vi "formatEvtDetails.vi"(8 "error in (no error)":errorcluster, 9 "evtName":string="move", 10 "evtDetailsString":string, 11 "TcpServer.lvclass":refnum<class "TcpServer.lvclass">) -> (0 "error out":errorcluster, 2 "jsonString":string, 3 "TcpServer.lvclass":refnum<class "TcpServer.lvclass">)   [LabVIEW 2018, in "TcpServer.lvclass"]
doc: "Prepare the Event with JSON format."
uses:
  TcpServer.lvclass
  <vilib>/Utility/error.llb/Error Cluster From Error Code.vi
  <vilib>/ErrorRing/Error Ring.xnode
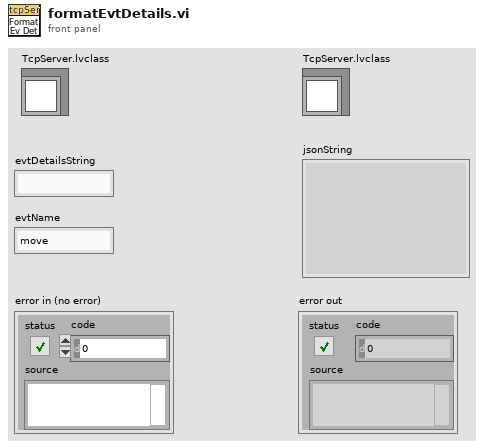
[diagram p1: front panel]
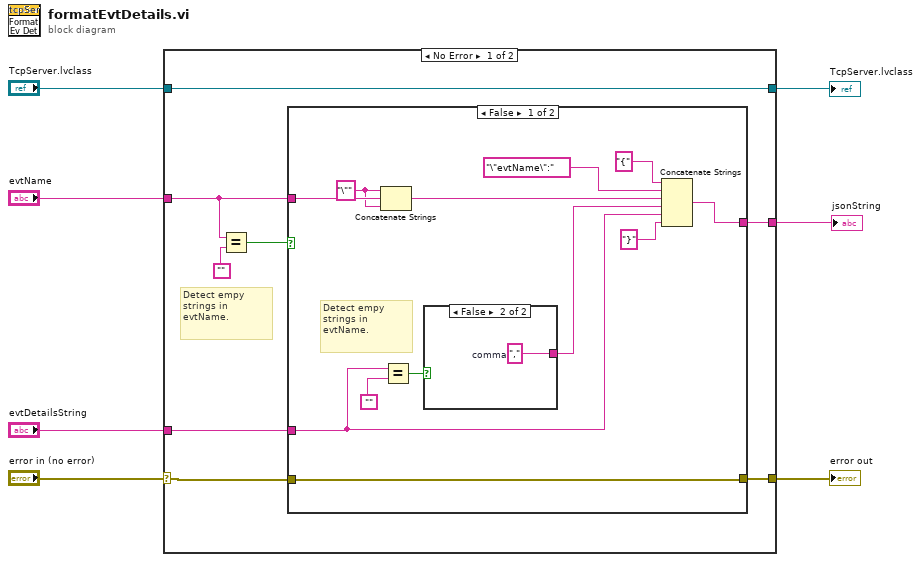
[diagram p0: block diagram]
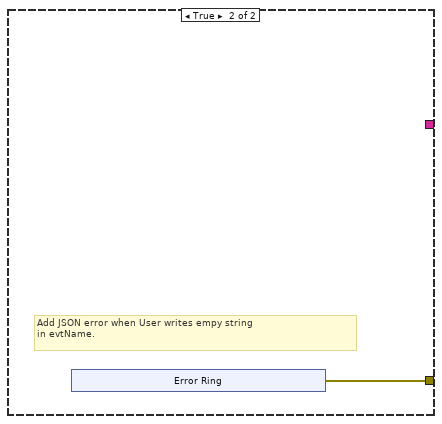
[diagram p3: hidden frame]
diagram:
  n1 = case shown="No Error" "error in (no error)" {
    selector: "error in (no error)" -> [w9 w34]
    tunnel: [w15 _] -> w1
    tunnel: "evtDetailsString" -> [w14 _]
    tunnel: "evtName" -> [w11 _]
    tunnel: "TcpServer.lvclass" -> [w13 w35]
    tunnel: [w13 w35] -> w3
    tunnel: [w8 w34] -> w2
    frame No Error {
      # "Detect empy\nstrings in \nevtName."
      n2 = Equal?(x=w11, y="") -> (x = y?=w10:bool)
      n3 = case shown="False" w10 {
        tunnel: [w27 _] -> w15
        tunnel: w14 -> [w25 _]
        tunnel: w11 -> [w26 _]
        tunnel: w9 -> [w16 _]
        tunnel: [w16 w29] -> w8
        frame False {
          w17 = "\"" ("string")
          # "Detect empy\nstrings in \nevtName."
          n4 = Concatenate Strings(w17, w26, w17) -> (w18:string)
          n5 = Equal?(x=w25, y="") -> (x = y?=w19:bool)
          n6 = case shown="False" w19 {
            tunnel: [_ w28] -> w23
            frame True {
            }
            frame False {
              w28 = ","  # comma
            }
          }
          n7 = Concatenate Strings("{" ("string"), "\"evtName\":", w18, w23, w25, "}" ("string")) -> (w27:string)
        }
        frame True {
          # "Add JSON error when User writes empy string\nin evtName."
          n8 = xnode "Error Ring"() -> ("error out"=w29:errorcluster)
        }
      }
    }
    frame Error {
    }
  }
  "jsonString" <- w1
  "error out" <- w2
  "TcpServer.lvclass" <- w3
